vi "CheckMapLimits.vi"(0 "object in":refnum<class "Battleship.lvclass">, 2 "MapLimits":T1, 5 "error in (no error)":errorcluster) -> (14 "object out":refnum<class "Battleship.lvclass">, 16 "WithinMapLimits?":bool, 19 "error out":errorcluster)   [LabVIEW 2015, in "Battleship.lvclass"]
doc: "Returns true if the ship is positioned within the size limits of the map."
uses:
  Battleship.lvclass
  TypDefs/Coordinates.ctl
  Battleship.lvclass/Battleship.ctl
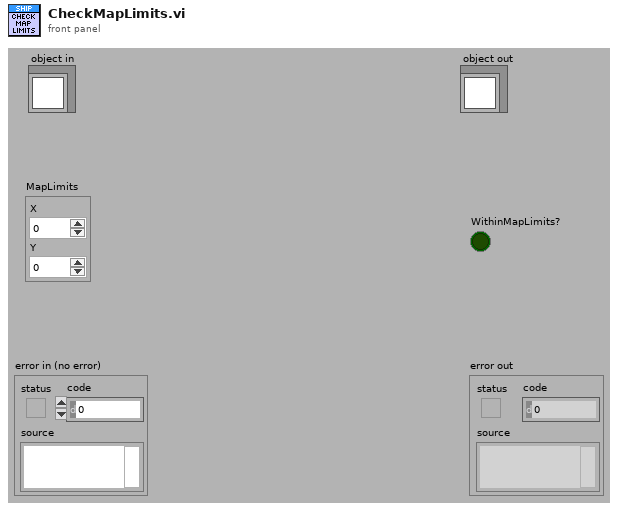
[diagram p1: front panel]
types:
  T1 = typedef "Coordinates.ctl" = cluster{"X":i32, "Y":i32}
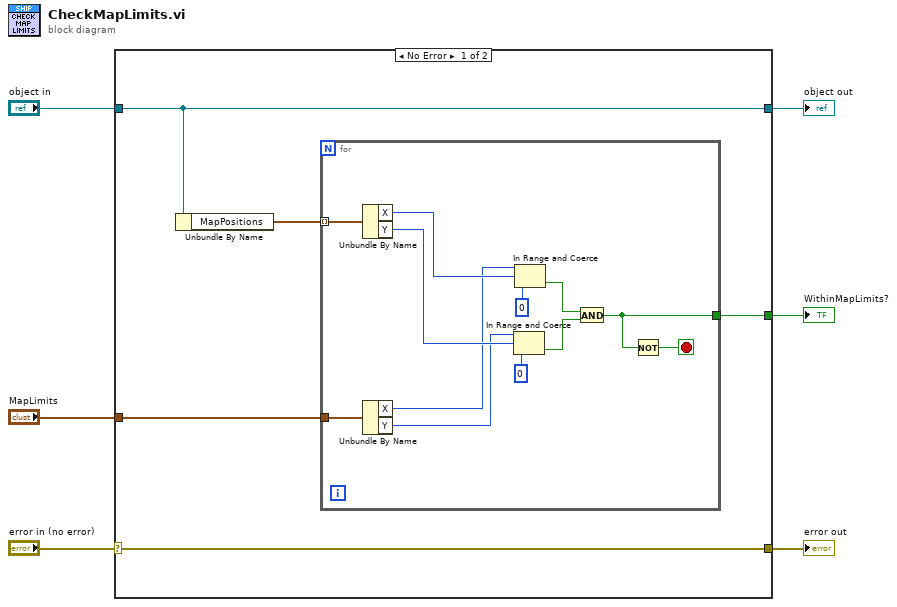
[diagram p0: block diagram]
diagram:
  n1 = case shown="No Error" "error in (no error)" {
    selector: "error in (no error)" -> [w11 w25]
    tunnel: [w11 w25] -> w5
    tunnel: [w10 w24] -> w3
    tunnel: "object in" -> [w10 w24]
    tunnel: "MapLimits" -> [w8 _]
    tunnel: [w7 _] -> w1
    frame No Error {
      n2 = Unbundle By Name(w10) -> ("MapPositions"=w9:T1[])
      n3 = for {
        tunnel: w9 -> [w23] mode=indexing
        tunnel: w8 -> [w22]
        tunnel: [w12] -> w7
        stop <- w13 stop-if-true
        n4 = Unbundle By Name(w23) -> ("X"=w21:i32, "Y"=w20:i32)
        n5 = Unbundle By Name(w22) -> ("X"=w17:i32, "Y"=w16:i32)
        n6 = In Range and Coerce(upper limit=w16, x=w20, lower limit=0) -> (In Range?=w14:bool)  [unwired: 1 out]
        n7 = In Range and Coerce(upper limit=w17, x=w21, lower limit=0) -> (In Range?=w15:bool)  [unwired: 1 out]
        n8 = And(x=w15, y=w14) -> (x .and. y?=w12:bool)
        n9 = Not(x=w12) -> (.not. x?=w13:bool)
      }
    }
    frame Error {
    }
  }
  "error out" <- w5
  "object out" <- w3
  "WithinMapLimits?" <- w1
